vi "(BASVR) Set Up Graph & Recorded Channel List.vi"(4 "error In":errorcluster, 7 "SUGRCL Input Cluster":T2) -> (0 "error out":errorcluster, 1 "SUGRCL Output Cluster":T1, 2 "Cleaned Channel List":string[](array[string]), 3 "X Scale.Display Format:Format":u8)   [LabVIEW 2023]
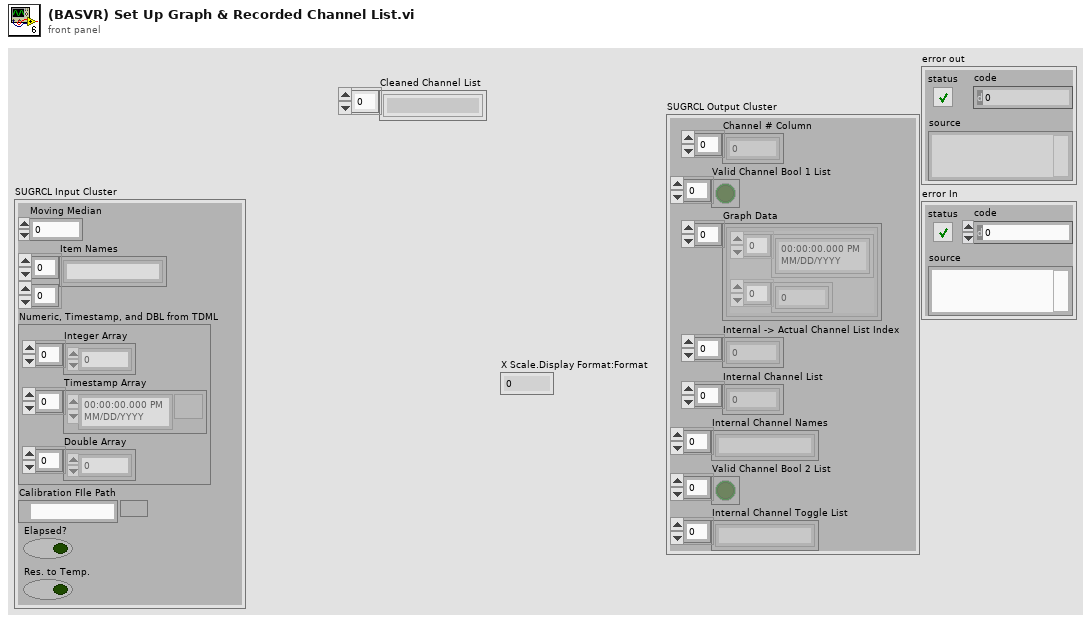
[diagram p1: front panel]
types:
  T1 = cluster{"Channel # Column":i32[], "Valid Channel Bool 1 List":bool[], "Graph Data":cluster{timestamp[], dbl[]}[], "Internal -> Actual Channel List Index":i32[], "Internal Channel List":i32[], "Internal Channel Names":string[], "Valid Channel Bool 2 List":bool[], "Internal Channel Toggle List":string[]}
  T2 = cluster{"Moving Median":u8, "Item Names":string[][], "Numeric, Timestamp, and DBL from TDML":cluster{"Integer Array":i32[], "Timestamp Array":timestamp[], "Double Array":dbl[]}, "Calibration FIle Path":path, "Elapsed?":bool, "Res. to Temp.":bool}
  T3 = cluster{"Integer Array":i32[], "Timestamp Array":timestamp[], "Double Array":dbl[]}
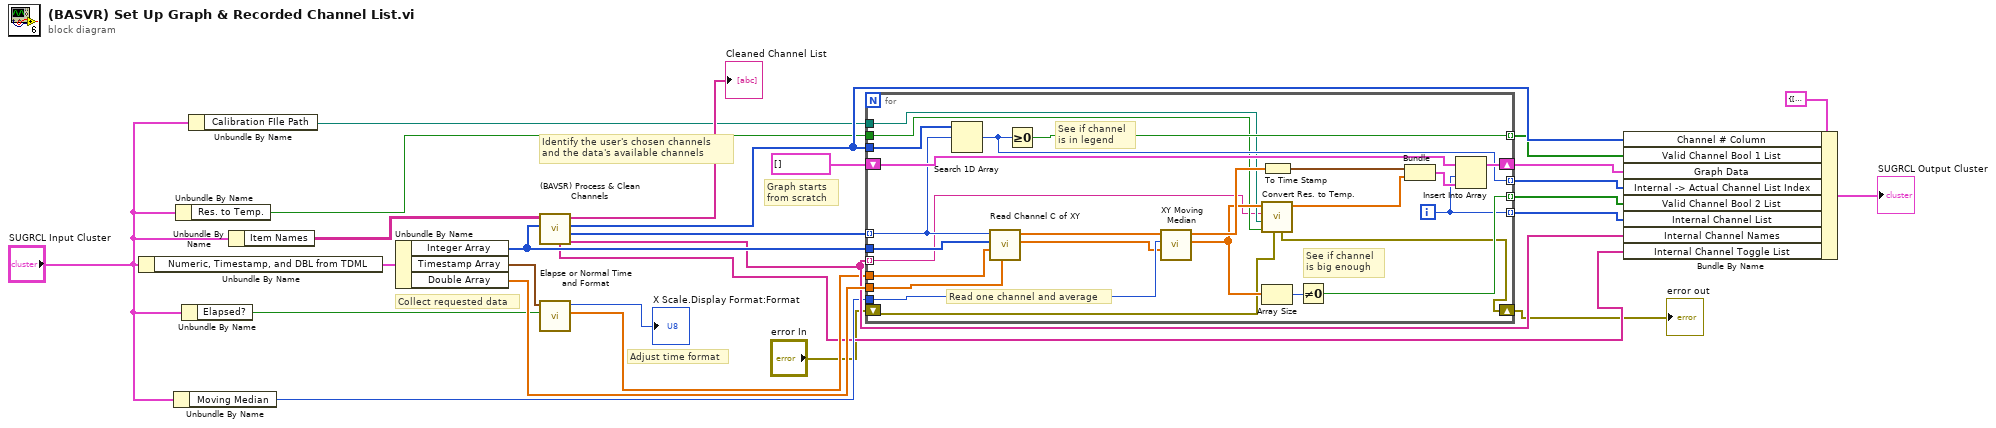
[diagram p0: block diagram]
diagram:
  # "Graph starts from scratch"
  # "Adjust time format"
  # "Identify the user's chosen channels and the data's available channels"
  # "Collect requested data"
  n1 = Unbundle By Name("SUGRCL Input Cluster") -> ("Numeric, Timestamp, and DBL from TDML"=w11:T3)
  n2 = Unbundle By Name("SUGRCL Input Cluster") -> ("Moving Median"=w9:u8)
  n3 = Unbundle By Name("SUGRCL Input Cluster") -> ("Res. to Temp."=w8:bool)
  n4 = Unbundle By Name("SUGRCL Input Cluster") -> ("Elapsed?"=w12:bool)
  n5 = Unbundle By Name("SUGRCL Input Cluster") -> ("Calibration FIle Path"=w7:path)
  n6 = Unbundle By Name("SUGRCL Input Cluster") -> ("Item Names"=w10:string[][])
  n7 = Unbundle By Name(w11) -> ("Integer Array"=w25:i32[], "Timestamp Array"=w26:timestamp[], "Double Array"=w27:dbl[])
  n8 = call "(BAVSR) Process & Clean Channels.vi"("C Array"=w25, "Channel Control & Legend"=w10) -> ("Relevant Channel Names"=w14:string[], "Relevant Channel List"=w24:i32[], "Channel # Column"=w20:i32[], "Cleaned Channel List"=→"Cleaned Channel List":string[], "Relevant Channel Label Toggles"=w4:string[])  [unwired: 5 in]
  n9 = call "Elapse or Normal Time and Format.vi"("Elapsed?"=w12, "Time Array"=w26) -> ("Time Array"=w5:dbl[], "X Scale.Display Format:Format"=→"X Scale.Display Format:Format":u8)  [unwired: 8 in]
  n10 = for {
    tunnel: w5 -> [w52]
    tunnel: w9 -> [w51]
    tunnel: w24 -> [w43] mode=indexing
    tunnel: w25 -> [w35]
    shift-right: [w45] -> w18
    shift-left: cluster{timestamp[], dbl[]}[] [] -> [w44]
    tunnel: w20 -> [w38]
    tunnel: [w39] -> w16 mode=indexing
    tunnel: [w36] -> w15 mode=indexing
    tunnel: [w41] -> w19 mode=indexing
    tunnel: [w40] -> w17 mode=indexing
    tunnel: w27 -> [w37]
    tunnel: w8 -> [w32]
    tunnel: w7 -> [w31]
    tunnel: w14 -> [w30] mode=indexing
    shift-right: [w28] -> w1
    shift-left: "error In" -> [w29]
    i -> [w36]
    # "See if channel is big enough"
    # "See if channel is in legend"
    # "Read one channel and average"
    n11 = Search 1D Array(1D array=w38, element=w43) -> (index of element=w40:i32)  [unwired: 1 in]
    n12 = call "Read Channel C of XY.vi"("Y"=w37, "X"=w52, "C"=w35, "Channel Chosen"=w43) -> ("Y"=w49:dbl[], "X"=w50:dbl[])  [unwired: 5 in, 1 out]
    n13 = Greater Or Equal To 0?(x=w40) -> (x >= 0?=w41:bool)
    n14 = call "XY Moving Median.vi"("Y Array"=w49, "Moving Median"=w51, "X Array"=w50) -> ("Y Array"=w34:dbl[], "X Array"=w48:dbl[])  [unwired: 6 in, 1 out]
    n15 = call "Convert Res. to Temp..vi"("error in"=w29, "Convert to Temp."=w32, "Calibration FIle"=w31, "Channel"=w30, "Y Array"=w34) -> ("Y Array"=w33:dbl[], "error out"=w28:errorcluster)  [unwired: 5 in]
    n16 = Array Size(array=w34) -> (size(s)=w42:i32)
    n17 = To Time Stamp(1:w48) -> (0:w46:timestamp[])
    n18 = Not Equal To 0?(x=w42) -> (x != 0?=w39:bool)
    n19 = Bundle(w46, "Y Array"=w33) -> (w47:cluster{timestamp[], "Y Array":dbl[]})  [unwired: 1 in]
    n20 = Insert Into Array(array=w44, index=w36, new element=w47) -> (w45:cluster{timestamp[], dbl[]}[])
  }
  "error out" <- w1
  n21 = Bundle By Name(cluster=T1 {"Channel # Column"=[], "Valid Channel Bool 1 List"=[], "Graph Data"=[], "Internal -> Actual Channel List Index"=[], "Internal Channel List"=[], "Internal Channel Names"=[], "Valid Channel Bool 2 List"=[], "Internal Channel Toggle List"=[]}, "Channel # Column"=w20, "Valid Channel Bool 1 List"=w19, "Graph Data"=w18, "Internal -> Actual Channel List Index"=w17, "Valid Channel Bool 2 List"=w16, "Internal Channel List"=w15, "Internal Channel Names"=w14, "Internal Channel Toggle List"=w4) -> (→"SUGRCL Output Cluster":T1)
